vi "PID_auto.vi"() -> (1 "output_ty":dbl, 2 "output_tx":dbl)   [LabVIEW 2020]
uses:
  Prog_Testes/GlobalVariables.vi
  <vilib>/functionblocks/Control/PID/PID.vi
  <vilib>/functionblocks/NI_FunctionBlock Libraries.lvlib
  <vilib>/functionblocks/FB Core/FB Core.xnode
panel:
  in  "Numeric":dbl
  in  "Numeric 2":dbl
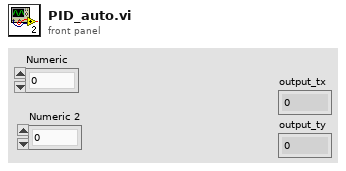
[diagram p1: front panel]
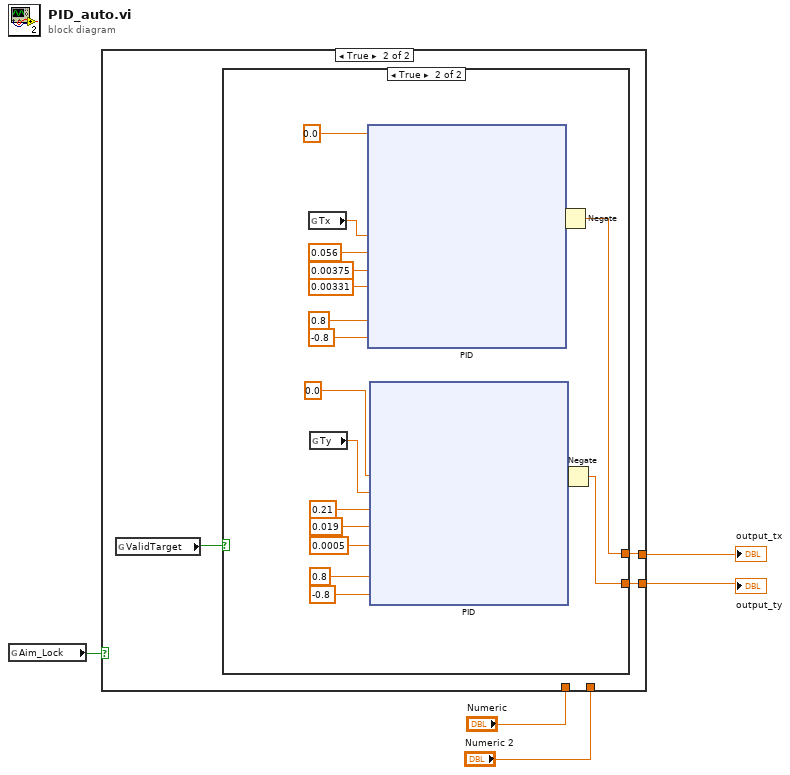
[diagram p0: block diagram]
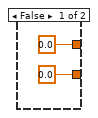
[diagram p3: hidden frame]
diagram:
  n1 = global read "GlobalVariables.vi" "Aim_Lock"() -> (w5:bool)
  n2 = case shown="True" w5 {
    tunnel: [w6 w9] -> w3
    tunnel: [w7 w10] -> w4
    tunnel: "Numeric" -> [w7 _]
    tunnel: "Numeric 2" -> [w6 _]
    frame False {
    }
    frame True {
      n3 = global read "GlobalVariables.vi" "ValidTarget"() -> (w8:bool)
      n4 = case shown="True" w8 {
        tunnel: [0.0 ("x+y") w30] -> w10
        tunnel: [0.0 ("x+y") w13] -> w9
        frame False {
        }
        frame True {
          n5 = global read "GlobalVariables.vi" "Tx"() -> (w28:dbl)
          n6 = global read "GlobalVariables.vi" "Ty"() -> (w16:dbl)
          n7 = xnode "PID"("setpoint"=0.0, "process variable"=w28, "proportional gain (Kc)"=0.056, "integral time (Ti, min)"=0.00375, "derivative time (Td, min)"=0.00331, "output high"=0.8, "output low"=-0.8) -> ("output"=w27:dbl)  [unwired: 2 in, 1 out]
          n8 = xnode "PID"("setpoint"=0.0, "process variable"=w16, "proportional gain (Kc)"=0.21, "integral time (Ti, min)"=0.019, "derivative time (Td, min)"=0.0005, "output high"=0.8, "output low"=-0.8) -> ("output"=w14:dbl)  [unwired: 2 in, 1 out]
          n9 = Negate(x=w27) -> (-x=w30:dbl)
          n10 = Negate(x=w14) -> (-x=w13:dbl)
        }
      }
    }
  }
  "output_tx" <- w4
  "output_ty" <- w3
